vi "Fixed PID.vi"() -> ()   [LabVIEW 2009, in "Varian Magnet.lvclass"]
uses:
  Varian Magnet.lvclass
  <vilib>/DAQmx/create/channels.llb/DAQmx Create Channel (AO-Voltage-Basic).vi
  <vilib>/DAQmx/write.llb/DAQmx Write (Analog DBL 1Chan 1Samp).vi
panel:
  out "Deriv":dynamicdata(graph)
  out "Integral":dynamicdata(graph)
  out "last 20 numbers":dbl[](array[numeric])
  in  "stop":bool
  out "Timer":dbl[unit]
  in  "start/stop":bool
  out "start time":dbl
  out "stop time":dbl
  in  "clear":bool
  out "running?":bool
  out "At Field":bool
  in  "Go to Field":bool
  in  "Field Desired Set":dbl[unit] min=0.0 max=1.2 step=0.1
  out "Current Field":dbl[unit](knob) caption="Tesla" scale=0.0..1.25
  out "Field Desired":dbl[unit] min=0.0 max=1.25 step=0.001
  out "Waveform Chart":dbl[unit](graph)
  in  "Control Voltage":dbl min=-9.0 max=9.0 format="%0.2f"
  # "Big Knob Ranges:\n0  :  0 T\n10:   0T -.3 T \n20:   0T - .55T\n30:   0T - .8 T \n40:   0T - 1.02T \n50: .05T- 1.13T \n60: .25T- >1.13T \n70: .45T- >1.13T"
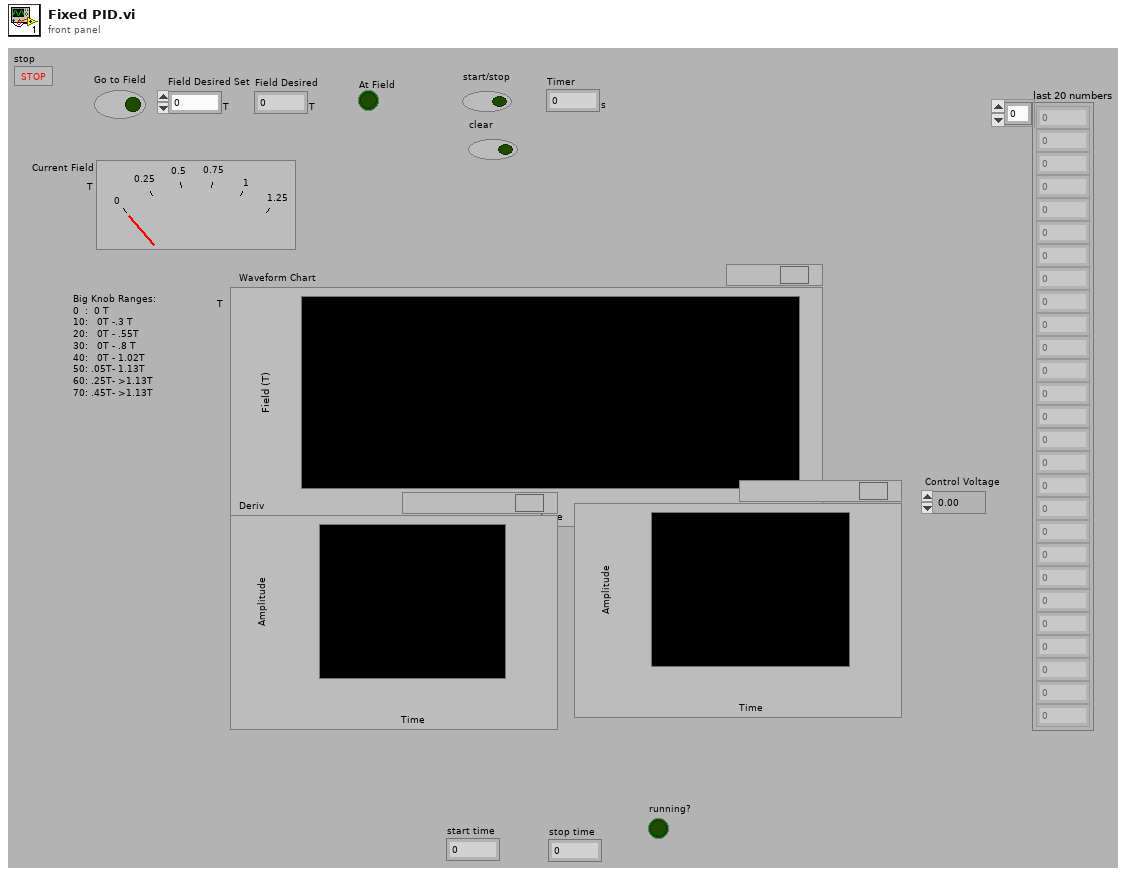
[diagram p1: front panel]
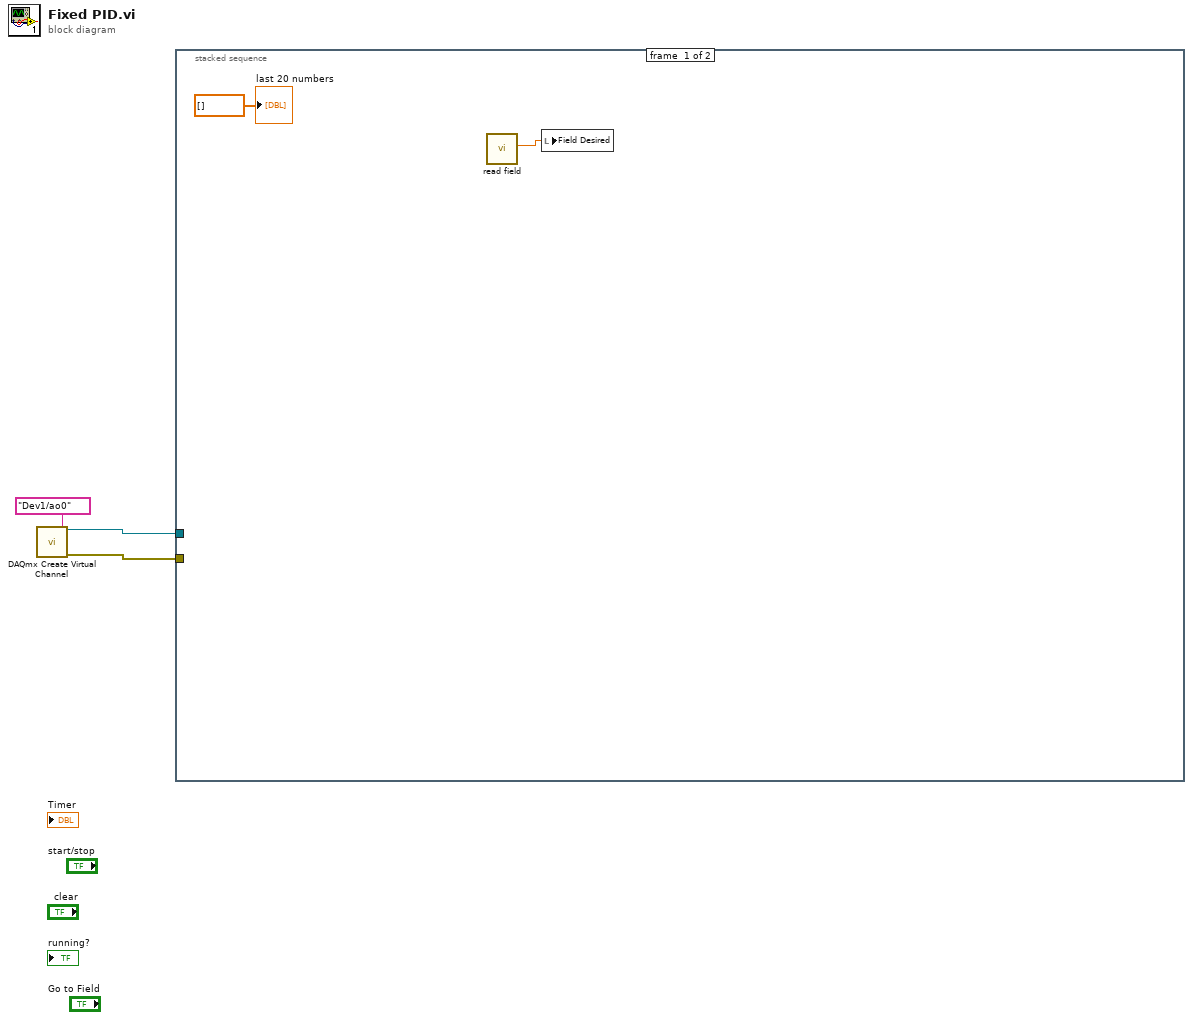
[diagram p0: block diagram]
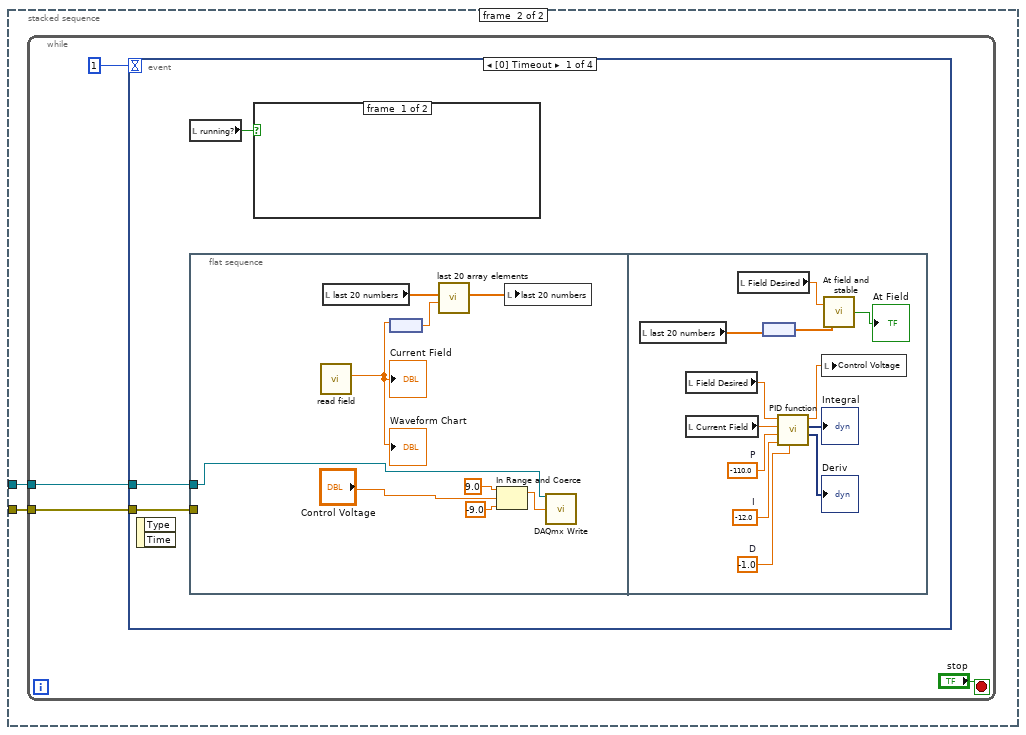
[diagram p2: hidden frame]
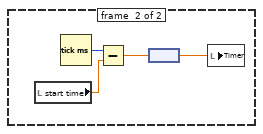
[diagram p3: hidden frame]
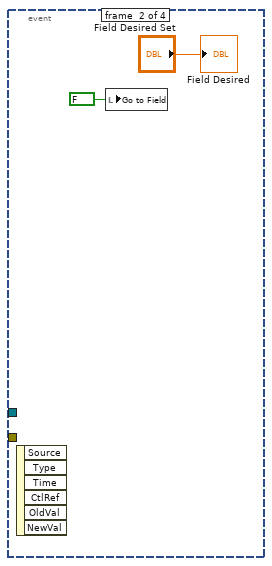
[diagram p4: hidden frame]
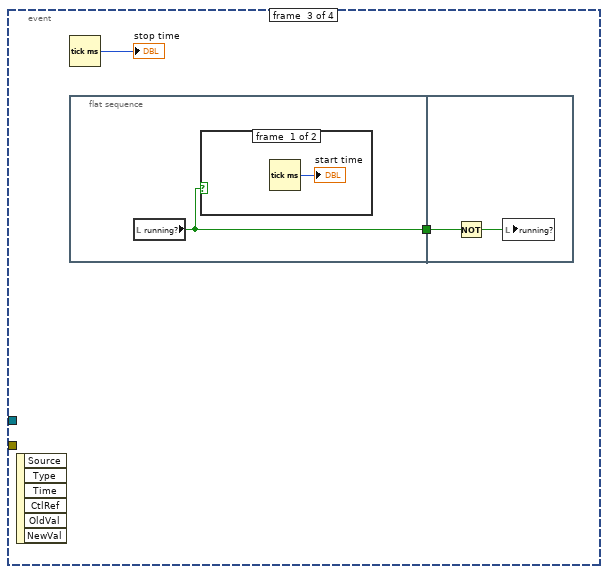
[diagram p5: hidden frame]
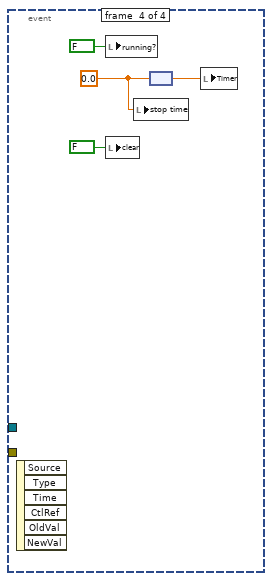
[diagram p7: hidden frame]
diagram:
  n1 = call-poly <vilib>:"DAQmx Create Virtual Channel.vi"("physical channels"=tag "Dev1/ao0") -> ("task out"=w2:refnum<k21>, "error out"=w3:errorcluster)  [unwired: 8 in, 5 out]
  n2 = stacked-sequence {
    tunnel: w3 -> [_ w7]
    tunnel: w2 -> [_ w6]
    frame #0 {
      n3 = call "read field.vi"() -> ("Current field (T)"=w4:dbl[unit])  [unwired: 1 in, 10 out]
      n4 = local write "Field Desired"(w4) -> ()
      "last 20 numbers" <- dbl[] [] ("last 20 field numbers")
    }
    frame #1 {
      n5 = while {
        tunnel: w7 -> [w9]
        tunnel: w6 -> [w10]
        stop <- "stop" stop-if-true
        n6 = event shown="[0] Timeout" {
          selector: _ -> [_ _ _ _]
          dyn-events: _ -> [_ _ _ _]
          timeout: 1 -> [_ _ _ _]
          tunnel: w10 -> [w13 _ _ _]
          tunnel: w9 -> [w12 _ _ _]
          event #0 {
            n7 = event-data() -> ()  [unwired: 3 out]
            n8 = local read "running?"() -> (w14:bool)
            n9 = flat-sequence {
              tunnel: w13 -> [w15]
              tunnel: w12 -> [_]
              frame #0 {
                n10 = call "read field.vi"() -> ("Current field (T)"=w21:dbl[unit])  [unwired: 1 in, 10 out]
                "Waveform Chart" <- w21
                "Current Field" <- w21
                n11 = local read "last 20 numbers"() -> (w23:dbl[])
                n12 = node(w21) -> (w20:dbl)
                n13 = call "last 20 array elements.vi"("number to be inserted at end"=w20, "input array"=w23) -> ("output array"=w22:dbl[])  [unwired: 9 out]
                n14 = In Range and Coerce(upper limit=9.0, x="Control Voltage", lower limit=-9.0) -> (coerced(x)=w19:dbl)  [unwired: 1 out]
                n15 = local write "last 20 numbers"(w22) -> ()
                n16 = call-poly <vilib>:"DAQmx Write.vi"("task/channels in"=w15, "data"=w19) -> ()  [unwired: 2 in, 12 out]
              }
              frame #1 {
                w31 = -12.0  # I
                w32 = -1.0  # D
                w30 = -110.0  # P
                n17 = local read "last 20 numbers"() -> (w34:dbl[])
                n18 = local read "Field Desired"() -> (w29:dbl[unit])
                n19 = local read "Current Field"() -> (w28:dbl[unit])
                n20 = local read "Field Desired"() -> (w35:dbl[unit])
                n21 = node(w34) -> (w24:dbl[unit][])
                n22 = call "PID function.vi"("D"=w32, "I"=w31, "P"=w30, "Current Field"=w28, "Field Desired"=w29) -> ("Deriv"=→"Deriv":dynamicdata, "Integral"=→"Integral":dynamicdata, "Numeric"=w27:dbl)  [unwired: 4 out]
                n23 = local write "Control Voltage"(w27) -> ()
                n24 = call "At field and stable.vi"("last 20 field numbers"=w24, "Desired field"=w35) -> ("At field and stable?"=→"At Field":bool)
              }
            }
            n25 = case shown="True" w14 {
              frame #0 {
              }
              frame #1 {
                n26 = local read "start time"() -> (w38:dbl)
                n27 = Tick Count (ms)() -> (millisecond timer value=w39:u32)
                n28 = Subtract(x=w39, y=w38) -> (x-y=w37:dbl)
                n29 = node(w37) -> (w36:dbl[unit])
                n30 = local write "Timer"(w36) -> ()
              }
            }
          }
          event #1 {
            n31 = event-data() -> ()  [unwired: 7 out]
            n32 = local write "Go to Field"(FALSE ("Go to Field")) -> ()
            "Field Desired" <- "Field Desired Set"
          }
          event #2 {
            n33 = event-data() -> ()  [unwired: 7 out]
            n34 = Tick Count (ms)() -> (millisecond timer value=→"stop time":u32)
            n35 = flat-sequence {
              tunnel: [w44] -> w43
              tunnel: w43 -> [w46]
              frame #0 {
                n36 = local read "running?"() -> (w44:bool)
                n37 = case shown="False" w44 {
                  frame #0 {
                    n38 = Tick Count (ms)() -> (millisecond timer value=→"start time":u32)
                  }
                  frame #1 {
                  }
                }
              }
              frame #1 {
                n39 = Not(x=w46) -> (.not. x?=w47:bool)
                n40 = local write "running?"(w47) -> ()
              }
            }
          }
          event #3 {
            w48 = 0.0 ("Time")
            n41 = event-data() -> ()  [unwired: 7 out]
            n42 = local write "running?"(FALSE ("running?")) -> ()
            n43 = local write "clear"(FALSE ("clear")) -> ()
            n44 = local write "stop time"(w48) -> ()
            n45 = node(w48) -> (w49:dbl[unit])
            n46 = local write "Timer"(w49) -> ()
          }
        }
      }
    }
  }
